vi "Read Vaisala Data.vi"(8 "error in (no error)":errorcluster, 11 "xData in":refnum<class "xData.lvclass">) -> (0 "error out":errorcluster, 2 "Vaisala Data":refnum<class "Single_Array.lvclass">[](array[class]), 3 "xData out":refnum<class "xData.lvclass">)   [LabVIEW 2014, in "xData.lvclass"]
uses:
  xData.lvclass
  reusable/Data/Array Data/Single 1-D/Single_Array.lvclass
  xData.lvclass/xData.ctl
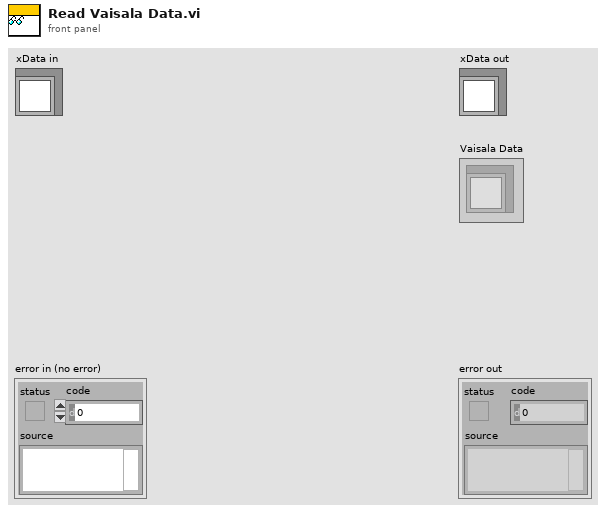
[diagram p1: front panel]
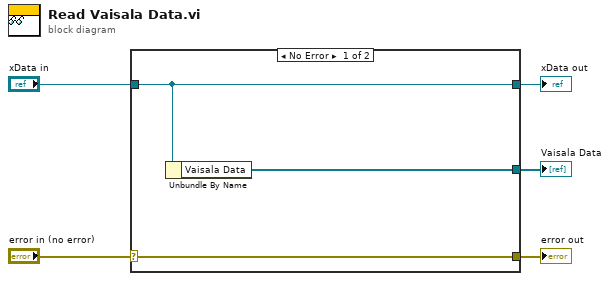
[diagram p0: block diagram]
diagram:
  n1 = case shown="No Error" "error in (no error)" {
    selector: "error in (no error)" -> [w8 w9]
    tunnel: [w8 w9] -> w4
    tunnel: [w7 w10] -> w2
    tunnel: "xData in" -> [w7 w10]
    tunnel: [w6 _] -> w1
    frame No Error {
      n2 = Unbundle By Name(w7) -> ("Vaisala Data"=w6:refnum<class "Single_Array.lvclass">[])
    }
    frame Error {
    }
  }
  "error out" <- w4
  "xData out" <- w2
  "Vaisala Data" <- w1
